vi "Write Input Data.vi"(10 "Input Data":T1={"Force Measured"=0.0, "Distance Data"={"Distance Measured"=1.0}} {"Distance Data"."Distance Measured" min=1.0 max=300.0 format="%.1f"; "Force Measured" min=-888.0 max=888.0 format="%.2f"}, 11 "Logger in":refnum<class "TestDataLog.lvclass">) -> (3 "Logger out":refnum<class "TestDataLog.lvclass">)   [LabVIEW 2015, in "TestDataLog.lvclass"]
uses:
  TestDataLog.lvclass
  Typedefs/InputData.ctl
  Typedefs/ForceDemand.ctl
  <userlib>/Common/Devices/DistanceGauge/Typedefs/Distance Data.ctl
  TestDataLog.lvclass/TestDataLog.ctl
  Typedefs/M1M3SSSTypedefs.lvlib
  <userlib>/Common/Devices/DistanceGauge/DistanceGauge.lvlib
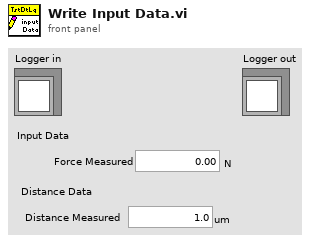
[diagram p1: front panel]
types:
  T1 = typedef "M1M3SSSTypedefs.lvlib/InputData.ctl" = cluster{"Force Measured":T2, "Distance Data":T3}
  T2 = typedef "M1M3SSSTypedefs.lvlib/ForceDemand.ctl" = dbl[unit]
  T3 = typedef "DistanceGauge.lvlib/Distance Data.ctl" = cluster{"Distance Measured":dbl[unit]}
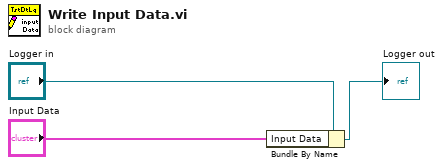
[diagram p0: block diagram]
diagram:
  n1 = Bundle By Name(cluster="Logger in", "Input Data"="Input Data") -> (→"Logger out":refnum<class "TestDataLog.lvclass">)
